vi "Analyze Data.vi"(8 "error in":errorcluster, 11 "nPAS in":refnum<class "nPAS.lvclass">) -> (0 "error out":errorcluster, 3 "nPAS out":refnum<class "nPAS.lvclass">)   [LabVIEW 2016, in "gPAS Library.lvlib" / "nPAS.lvclass"]
doc: "This is the core routine for PAS microphone data analysis. Here, the microphone data is retrieved from each of the cells. In both cases, the time domain signal will be transformed to the frequency domain. If the speaker is on (<B>Spk Pos</B> == TRUE), then the frequency domain signal will be squared to obtain the power and a Lorentzian will be fit to the data to retrieve the resonant characteristics of the cell. If the speaker is off (<B>Spk Pos</B> == FALSE), then the amplitude will be used to calculate the integrated area of the signal. In every case, the implementation has the ability to decimate the data for transmission of the waveforms over a network line."
uses:
  nPAS.lvclass
  C:/Program Files (x86)/National Instruments/LabVIEW 2016/vi.lib/MSR Consulting, LLC/General Reuse/Instrument/Instrument.lvclass
  <vilib>/MSR Consulting, LLC/General Reuse/PAS/Data/Main/PAS Data.lvclass
  C:/Program Files (x86)/National Instruments/LabVIEW 2016/vi.lib/MSR Consulting, LLC/General Reuse/Data/Data.lvclass
  <vilib>/MSR Consulting, LLC/General Reuse/Instrument/Instrument.lvclass/Instrument.ctl
  <vilib>/MSR Consulting, LLC/General Reuse/Instrument/Read Data Notifier.vi
  <vilib>/MSR Consulting, LLC/General Reuse/Instrument/Read Data.vi
  <vilib>/MSR Consulting, LLC/General Reuse/PAS/Main/PAS.lvclass
  <vilib>/MSR Consulting, LLC/General Reuse/Data/Data.lvclass
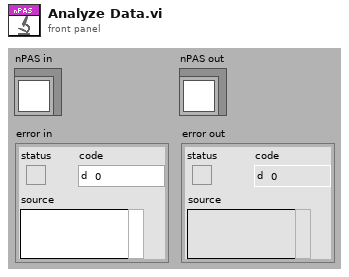
[diagram p1: front panel]
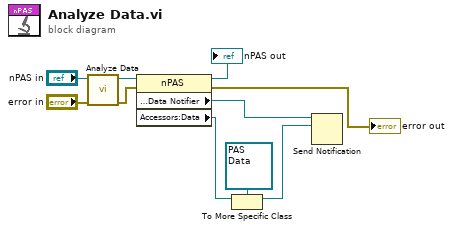
[diagram p0: block diagram]
diagram:
  n1 = call-parent "Analyze Data.vi"("error in"="error in", "PAS in"="nPAS in") -> ("error out"=w5:errorcluster, "PAS out"=w6:refnum<class "nPAS.lvclass">)  [unwired: 8 in]
  n2 = property class="nPAS"(reference=w6, error in=w5) -> (reference out=→"nPAS out":refnum<class "nPAS.lvclass">, error out=→"error out":errorcluster, "Accessors:Data Notifier"=w2:refnum<notifier>, "Accessors:Data"=w3:refnum<class "Data.lvclass">)
  n3 = To More Specific Class(target class=refnum<class "PAS Data.lvclass"> refnum ("PAS Library.lvlib:PAS Data"), reference=w3) -> (specific class reference=w1:refnum<class "PAS Data.lvclass">)  [unwired: 1 in, 1 out]
  n4 = Send Notification(notification=w1, notifier=w2) -> ()  [unwired: 1 in, 2 out]
